vi "Close Caller.vi"(8 "error in (no error)":errorcluster, 10 "Caller":T1, 11 "Open Close Logic in":refnum<class "Open Close Logic.lvclass">) -> (0 "error out":errorcluster, 2 "Close Nested":T1[](array[typedef]), 3 "Open Close Logic out":refnum<class "Open Close Logic.lvclass">)   [LabVIEW 2020, in "Form Server Interfaces.lvlib" / "Open Close Logic.lvclass"]
uses:
  Open Close Logic.lvclass
  Form ID.ctl
  Form Server Interfaces.lvlib
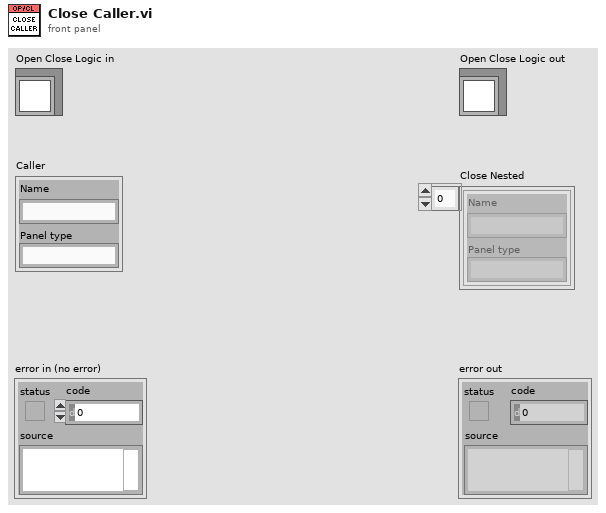
[diagram p1: front panel]
types:
  T1 = typedef "Form Server Interfaces.lvlib/Form ID.ctl" = cluster{"Name":string, "Panel type":string}
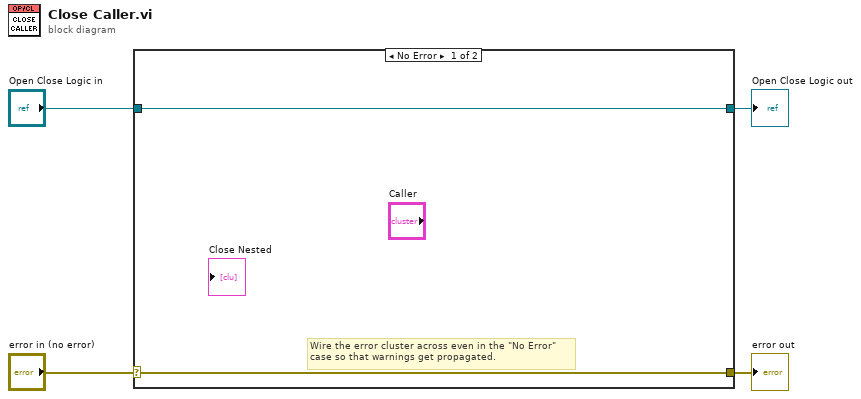
[diagram p0: block diagram]
diagram:
  n1 = case shown="No Error" "error in (no error)" {
    selector: "error in (no error)" -> [w5 w8]
    tunnel: [w5 w8] -> w3
    tunnel: [w6 w7] -> w1
    tunnel: "Open Close Logic in" -> [w6 w7]
    frame No Error {
      # "Wire the error cluster across even in the \"No Error\"\ncase so that warnings get propagated."
    }
    frame Error {
    }
  }
  "error out" <- w3
  "Open Close Logic out" <- w1
